vi "After Launch Init Core.vi"(8 "error in (no error)":errorcluster, 11 "CS++BaseActor in":refnum<class "CS++BaseActor.lvclass">) -> (0 "error out":errorcluster, 3 "CS++BaseActor out":refnum<class "CS++BaseActor.lvclass">)   [LabVIEW 2015, in "CS++BaseActor.lvlib" / "CS++BaseActor.lvclass"]
doc: "Use <b>Pre Launch init.vi</b> method only for sanity checks that are supposed to prevent the actor from launching if they fail. Use <B>this</B> method instead to initialize unique resources that must be released during the <b>Stop Core.vi</b> method. A corresponding high priority message will become dispatched before the <B>Actor Framework.lvlib:Actor.lvclass.Actor Core.vi</b> is called.\n\n<b>Derived classed should call the parent methode first</b> and their own initialization code after.\n\nRefer also to the ongoing discussion at https://decibel.ni.com/content/message/57394#57394."
uses:
  CS++BaseActor.lvclass
  Classes/CS++ProcessVariables/ProcessVariable/PV.lvclass
  CS++BaseActor.lvclass/CS++BaseActor.ctl
  Classes/CS++ProcessVariables/ProcessVariable/PV.lvclass/PV.ctl
  Classes/CS++ProcessVariables/ProcessVariable/Write Data.vi
  Classes/CS++ProcessVariables/ProcessVariable/Write Timestamp.vi
  Classes/CS++ProcessVariables/PVConnection/PVConnection.lvclass
  Libraries/Utilities/CS++Utilities.lvlib
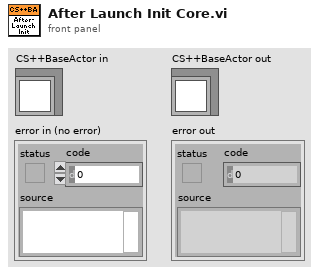
[diagram p1: front panel]
types:
  T1 = cluster{"Read Access":enum8{"Allowed", "Required", "None"}, "Write Access":enum8{"Allowed", "Required", "None"}}
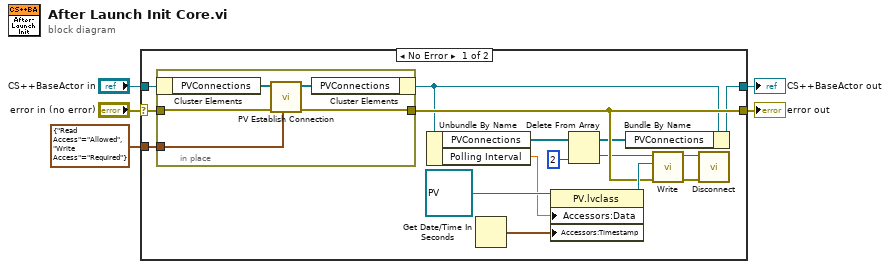
[diagram p0: block diagram]
diagram:
  n1 = case shown="No Error" "error in (no error)" {
    selector: "error in (no error)" -> [w20 w28]
    tunnel: [w13 w28] -> w4
    tunnel: [w8 w27] -> w2
    tunnel: "CS++BaseActor in" -> [w21 w27]
    tunnel: T1 {"Read Access"=enum."Allowed", "Write Access"=enum."Required"} ("Access (R/W allowed)") -> [w6 _]
    frame No Error {
      n2 = in-place {
        in-place-border: [w23] -> w13
        in-place-border: w20 -> [w24]
        in-place-border: w6 -> [w22]
        n3 = in-place-cluster #1(w21) -> ("PVConnections"=w26:refnum<class "PVConnection.lvclass">[])
        n4 = call "PV Establish Connection.vi"("Access (R/W allowed)"=w22, "Error In"=w24, "PVConnections in"=w26) -> ("Error Out"=w23:errorcluster, "PVConnections out"=w25:refnum<class "PVConnection.lvclass">[])  [unwired: 7 in]
        n5 = in-place-cluster #1("PVConnections"=w25) -> (w9:refnum<class "CS++BaseActor.lvclass">)
      }
      n6 = Unbundle By Name(w9) -> ("PVConnections"=w12:refnum<class "PVConnection.lvclass">[], "Polling Interval"=w17:dbl[unit])
      n7 = Get Date/Time In Seconds() -> (seconds since 1Jan1904=w16:timestamp)
      n8 = property class="PV.lvclass"(reference=refnum<class "PV.lvclass"> refnum ("CS++ProcessVariables.lvlib:PV.lvclass"), "Accessors:Data"=w17, "Accessors:Timestamp"=w16) -> (reference out=w18:refnum<class "PV.lvclass">)  [unwired: 1 in, 1 out]
      n9 = Delete From Array(array=w12, index=2) -> (deleted portion=w10:refnum<class "PVConnection.lvclass">, array with subset deleted=w7:refnum<class "PVConnection.lvclass">[])  [unwired: 1 in]
      n10 = Bundle By Name(cluster=w9, "PVConnections"=w7) -> (w8:refnum<class "CS++BaseActor.lvclass">)
      n11 = call "Write.vi"("error in (no error)"=w13, "PV"=w18, "PVConnection in"=w10) -> ("error out"=w14:errorcluster, "PVConnection out"=w15:refnum<class "PVConnection.lvclass">)  [unwired: 7 in]
      n12 = call "Disconnect.vi"("error in (no error)"=w14, "PVConnection in"=w15) -> ()  [unwired: 8 in, 2 out]
    }
    frame Error {
    }
  }
  "error out" <- w4
  "CS++BaseActor out" <- w2
